vi "Setup subWorker - FP_Emulator.vi"(8 "error in":errorcluster, 11 "Device Manager in":refnum<class "Device Manager.lvclass">) -> (0 "error out":errorcluster, 3 "Device Manager out":refnum<class "Device Manager.lvclass">)   [LabVIEW 2017, in "Device Manager.lvclass"]
doc: "This VI sets up the framework parameters of a statically-linked subWorker."
uses:
  Device Manager.lvclass
  Device Manager.lvclass/Device Manager.ctl
  Front Panel Emulator/Front Panel Emulator.lvclass
  C:/Program Files (x86)/National Instruments/LabVIEW 2017/vi.lib/addons/_Workers/Library/Classes/Worker/Worker.lvclass
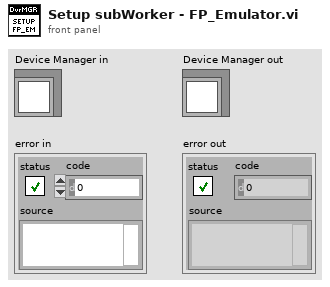
[diagram p1: front panel]
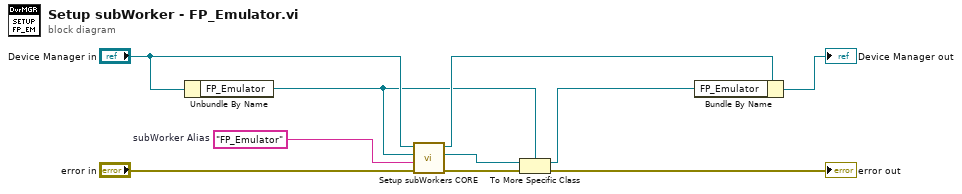
[diagram p0: block diagram]
diagram:
  w6 = "FP_Emulator"  # subWorker Alias
  n1 = Unbundle By Name("Device Manager in") -> ("FP_Emulator"=w3:refnum<class "Front Panel Emulator.lvclass">)
  n2 = call-dynamic "Setup subWorkers CORE.vi"("error in"="error in", "subWorker Alias"=w6, "subWorker"=w3, "Worker"="Device Manager in") -> ("error out"=w5:errorcluster, "subWorker out"=w1:refnum<class "Worker.lvclass">, "Worker out"=w8:refnum<class "Device Manager.lvclass">)  [unwired: 5 in]
  n3 = To More Specific Class(target class=w3, reference=w1, error in=w5) -> (specific class reference=w2:refnum<class "Front Panel Emulator.lvclass">, error out=→"error out":errorcluster)
  n4 = Bundle By Name(cluster=w8, "FP_Emulator"=w2) -> (→"Device Manager out":refnum<class "Device Manager.lvclass">)
